vi "listen for stop or shutdown.vi"(8 "error in (no error)":errorcluster) -> (0 "error out":errorcluster, 3 "Shutdown command received?":bool)   [LabVIEW 2012, in "GFG library.lvlib"]
uses:
  GFG/GFG library.lvlib
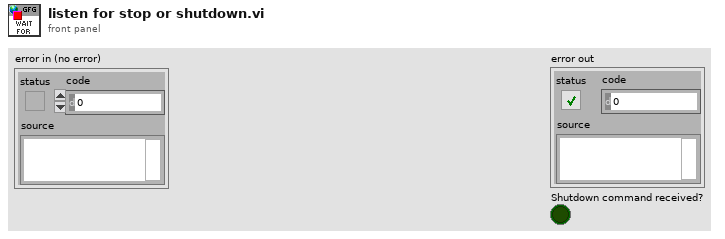
[diagram p1: front panel]
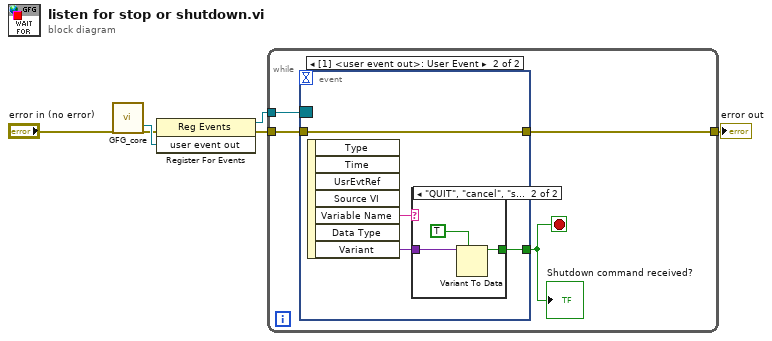
[diagram p0: block diagram]
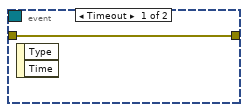
[diagram p2: hidden frame]
diagram:
  n1 = call "GFG_core.vi"("error in (no error)"="error in (no error)") -> ("user event out"=w5:refnum<user-event>, "error out"=w4:errorcluster)  [unwired: 12 in, 5 out]
  n2 = register-events(error in=w4, w5) -> (reference out=w6:refnum<event-registration>, error out=w2:errorcluster)  [unwired: 1 in]
  n3 = while {
    tunnel: w6 -> [w10]
    tunnel: w2 -> [w8]
    tunnel: [w7] -> w1
    stop <- w9 stop-if-true
    n4 = event shown="[1] <user event out>: User Event" {
      selector: w10 -> [_ _]
      dyn-events: _ -> [_ _]
      timeout: _ -> [_ _]
      tunnel: [_ w13] -> w9
      tunnel: w8 -> [w11 w12]
      tunnel: [w11 w12] -> w7
      event Timeout {
        n5 = event-data() -> ()  [unwired: 1 in, 2 out]
      }
      event User Event {
        n6 = event-data() -> ("Variable Name"=w15:string, "Variant"=w14:variant)  [unwired: 1 in, 5 out]
        n7 = case shown="\"QUIT\", \"cancel\", \"shutdown\"" w15 {
          tunnel: w14 -> [_ w18]
          tunnel: [_ w16] -> w13
          frame "False", Default {
          }
          frame "QUIT", "cancel", "shutdown" {
            n8 = Variant To Data(type=TRUE ("want seconds? (F)"), Variant=w18) -> (data=w16:bool)  [unwired: 1 in, 1 out]
          }
        }
      }
    }
    "Shutdown command received?" <- w9
  }
  "error out" <- w1
